vi "CAN_controlMode.vi"(8 "error in (no error)":errorcluster, 10 "Control Mode":T2) -> (0 "error out":errorcluster, 3 "output cluster":T4)   [LabVIEW 2009, in "OWNCAN.lvlib"]
uses:
  OWNCAN.lvlib
  CAN.lvlib
  CAN/SubVIs/CAN Jaguar Control Mode.ctl
  CAN/SubVIs/CAN Jaguar Ref.ctl
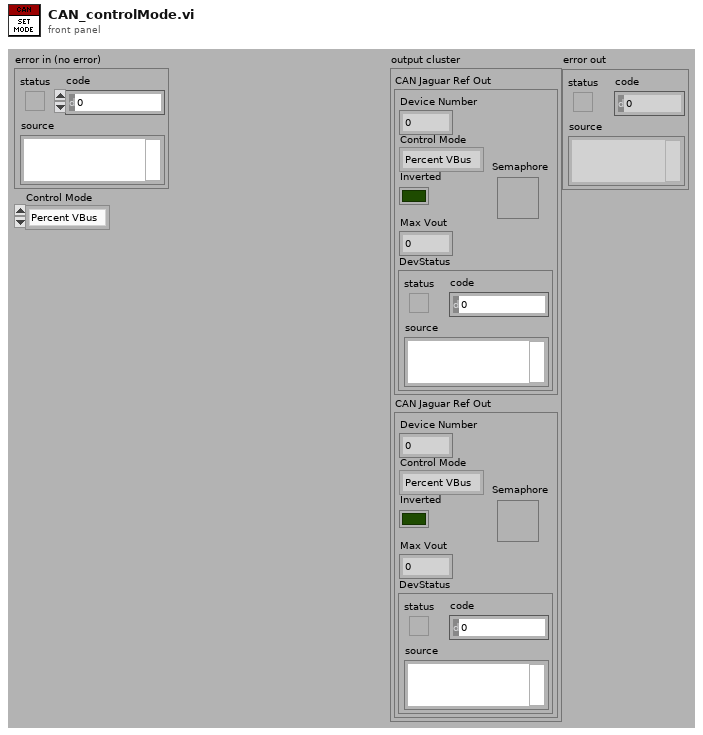
[diagram p1: front panel]
types:
  T1 = typedef "CAN.lvlib/CAN Jaguar Ref.ctl" = cluster{"Device Number":u8, "Control Mode":T2, "Inverted":bool, "Semaphore":T3, "Max Vout":dbl, "DevStatus":errorcluster}
  T2 = typedef "CAN.lvlib/CAN Jaguar Control Mode.ctl" = enum16{"Percent VBus", "Speed", "Position", "Current"}
  T3 = typedef "Semaphore RefNum" = refnum<k1>
  T4 = cluster{"CAN Jaguar Ref Out":T1, "CAN Jaguar Ref Out":T1}
  T5 = cluster{"PID Position":cluster{"P":dbl, "I":dbl, "D":dbl}, "PID Position 2":cluster{"P":dbl, "I":dbl, "D":dbl}}
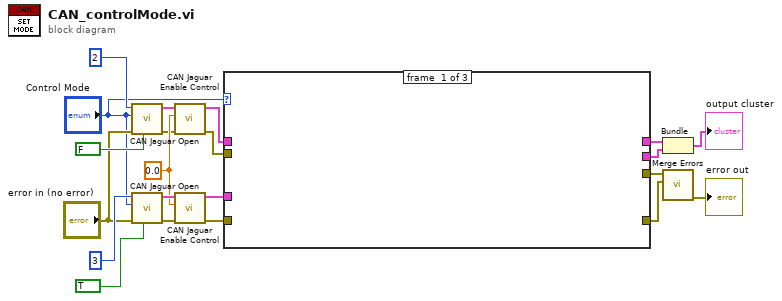
[diagram p0: block diagram]
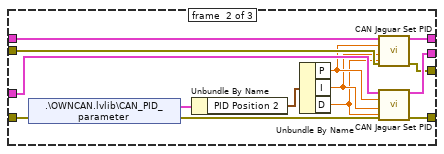
[diagram p2: hidden frame]
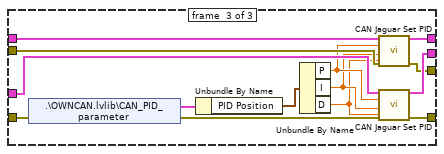
[diagram p3: hidden frame]
diagram:
  w14 = 0.0 ("Encoder Initial Position")
  n1 = call "CAN Jaguar Open.vi"("Inverted"=FALSE, "error in (no error)"="error in (no error)", "Control Mode"="Control Mode", "Device Number"=u8 2) -> ("error out"=w13:errorcluster, "CAN Jaguar Ref Out"=w11:T1)  [unwired: 6 in]
  n2 = call "CAN Jaguar Open.vi"("Inverted"=TRUE, "error in (no error)"="error in (no error)", "Control Mode"="Control Mode", "Device Number"=u8 3) -> ("error out"=w12:errorcluster, "CAN Jaguar Ref Out"=w15:T1)  [unwired: 6 in]
  n3 = call "CAN Jaguar Enable Control.vi"("error in (no error)"=w13, "Encoder Initial Position"=w14, "CAN Jaguar Ref"=w11) -> ("error out"=w8:errorcluster, "CAN Jaguar Ref Out"=w7:T1)  [unwired: 7 in]
  n4 = call "CAN Jaguar Enable Control.vi"("error in (no error)"=w12, "Encoder Initial Position"=w14, "CAN Jaguar Ref"=w15) -> ("error out"=w5:errorcluster, "CAN Jaguar Ref Out"=w6:T1)  [unwired: 7 in]
  n5 = case shown="\"Position\"" "Control Mode" {
    tunnel: w8 -> [_ w35 w49]
    tunnel: w7 -> [_ w34 w48]
    tunnel: w6 -> [_ w33 w47]
    tunnel: w5 -> [_ w27 w41]
    tunnel: [_ w32 w46] -> w4
    tunnel: [_ w31 w45] -> w3
    tunnel: [_ w30 w44] -> w2
    tunnel: [_ w29 w43] -> w1
    frame #0 {
    }
    frame #1 {
      n6 = shared-variable ".\\OWNCAN.lvlib\\CAN_PID_parameter"(error in=w27) -> (w28:T5, error out=w26:errorcluster)
      n7 = Unbundle By Name(w28) -> ("PID Position 2"=w25:cluster{"P":dbl, "I":dbl, "D":dbl})
      n8 = Unbundle By Name(w25) -> ("P"=w24:dbl, "I"=w23:dbl, "D"=w22:dbl)
      n9 = call "CAN Jaguar Set PID.vi"("CAN Jaguar Ref"=w34, "P"=w24, "I"=w23, "D"=w22, "error in (no error)"=w35) -> ("CAN Jaguar Ref Out"=w31:T1, "error out"=w30:errorcluster)  [unwired: 9 in]
      n10 = call "CAN Jaguar Set PID.vi"("CAN Jaguar Ref"=w33, "P"=w24, "I"=w23, "D"=w22, "error in (no error)"=w26) -> ("CAN Jaguar Ref Out"=w32:T1, "error out"=w29:errorcluster)  [unwired: 9 in]
    }
    frame #2 {
      n11 = shared-variable ".\\OWNCAN.lvlib\\CAN_PID_parameter"(error in=w41) -> (w42:T5, error out=w40:errorcluster)
      n12 = Unbundle By Name(w42) -> ("PID Position"=w39:cluster{"P":dbl, "I":dbl, "D":dbl})
      n13 = Unbundle By Name(w39) -> ("P"=w38:dbl, "I"=w37:dbl, "D"=w36:dbl)
      n14 = call "CAN Jaguar Set PID.vi"("CAN Jaguar Ref"=w48, "P"=w38, "I"=w37, "D"=w36, "error in (no error)"=w49) -> ("CAN Jaguar Ref Out"=w45:T1, "error out"=w44:errorcluster)  [unwired: 9 in]
      n15 = call "CAN Jaguar Set PID.vi"("CAN Jaguar Ref"=w47, "P"=w38, "I"=w37, "D"=w36, "error in (no error)"=w40) -> ("CAN Jaguar Ref Out"=w46:T1, "error out"=w43:errorcluster)  [unwired: 9 in]
    }
  }
  n16 = Bundle("CAN Jaguar Ref Out"=w3, "CAN Jaguar Ref Out"=w4) -> (→"output cluster":T4)  [unwired: 1 in]
  n17 = call <vilib>:"Merge Errors.vi"("error in 2 (no error)"=w1, "error in 1 (no error)"=w2) -> ("error out"=→"error out":errorcluster)  [unwired: 5 in]
